vi "file loading.vi"() -> ()   [LabVIEW 2018]
panel:
  out "Error Out":errorcluster
  out "LoadFile":bool
  in  "File Path Control":path
  in  "?":refnum<k7>(container)
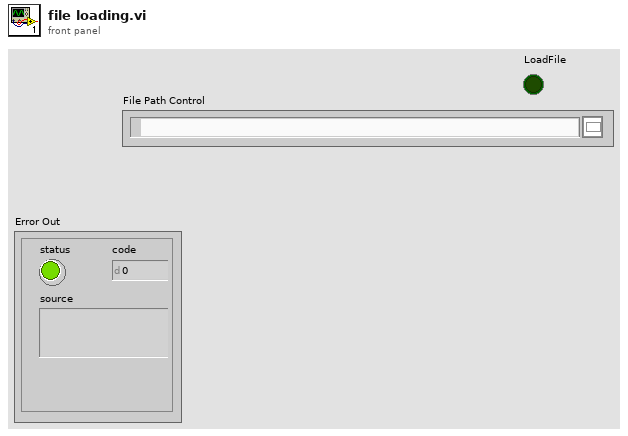
[diagram p1: front panel]
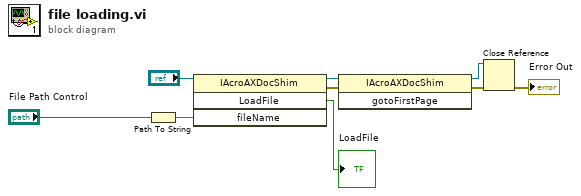
[diagram p0: block diagram]
diagram:
  n1 = Path To String(path="File Path Control") -> (string=w7:string)
  n2 = invoke class="IAcroAXDocShim" method="LoadFile"(reference="?", "fileName"=w7) -> (reference out=w5:refnum<k7>, error out=w2:errorcluster, "LoadFile"=→"LoadFile":bool)  [unwired: 2 in, 1 out]
  n3 = invoke class="IAcroAXDocShim" method="gotoFirstPage"(reference=w5, error in=w2) -> (reference out=w4:refnum<k7>, error out=w3:errorcluster)  [unwired: 1 in, 1 out]
  n4 = Close Reference(reference=w4, error in (no error)=w3) -> (error out=→"Error Out":errorcluster)
